vi "Common Device Queue Messenger.vi"(2 "Common Action":T1=enum."Open Front Panel", 7 "Notifier Name":string="Not a Name", 13 "Specific Action":string="No Action") -> (8 "Notifier Name":string)   [LabVIEW 2016]
uses:
  Common Device Controls/Common Device Actions.ctl
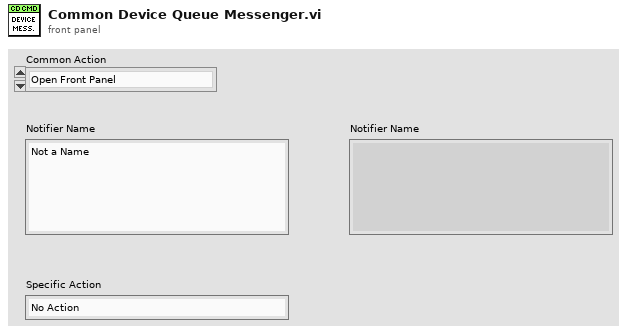
[diagram p1: front panel]
types:
  T1 = typedef "Common Device Actions.ctl" = enum16{"Specific Action", "Open Front Panel", "Close Front Panel", "Quit", "Quit All"}
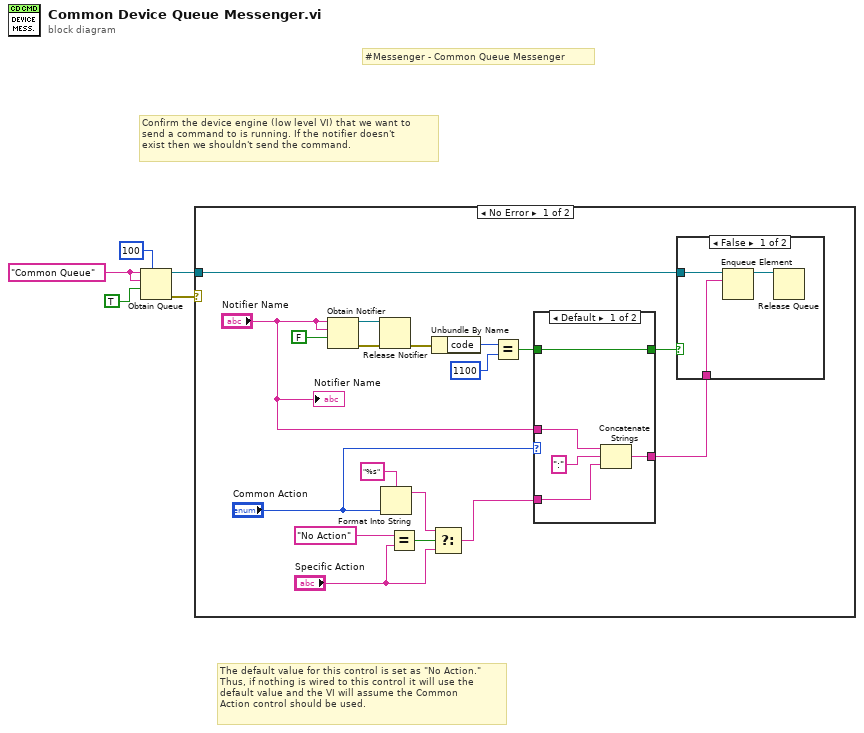
[diagram p0: block diagram]
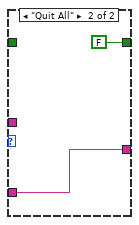
[diagram p3: hidden frame]
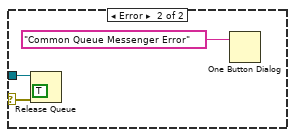
[diagram p4: hidden frame]
diagram:
  w1 = "Common Queue" ("Unique Notifier Name")
  # "Confirm the device engine (low level VI) that we want to\nsend a command to is running. If the notifier doesn't\nexist then we shouldn't send the command."
  # "The default value for this control is set as \"No Action.\"\nThus, if nothing is wired to this control it will use the\ndefault value and the VI will assume the Common\nAction control should be used."
  # "#Messenger - Common Queue Messenger"
  n1 = Obtain Queue(max queue size (-1, unlimited)=100, name (unnamed)=w1, element data type=w1, create if not found? (T)=TRUE) -> (queue out=w5:refnum<queue>, error out=w4:errorcluster)  [unwired: 1 in, 1 out]
  n2 = case shown="No Error" w4 {
    selector: w4 -> [_ w35]
    tunnel: w5 -> [w10 w37]
    frame No Error {
      n3 = Obtain Notifier(name (unnamed)="Notifier Name", notification data type="Notifier Name", create if not found? (T)=FALSE) -> (notifier out=w21:refnum<notifier>, error out=w22:errorcluster)  [unwired: 1 in, 1 out]
      n4 = Release Notifier(notifier=w21, error in (no error)=w22) -> (error out=w23:errorcluster)  [unwired: 1 in, 2 out]
      n5 = Format Into String(format string="%s", "Common Action") -> (resulting string=w16:string)  [unwired: 2 in, 1 out]
      n6 = Equal?(x="No Action" ("Unique Notifier Name"), y="Specific Action") -> (x = y?=w15:bool)
      n7 = Unbundle By Name(w23) -> ("code"=w20:i32)
      n8 = Select(t=w16, s=w15, f="Specific Action") -> (s? t:f=w12:string)
      n9 = Equal?(x=w20, y=1100) -> (x = y?=w7:bool)
      n10 = case shown="Default" "Common Action" {
        tunnel: [w31 w33] -> w9
        tunnel: w12 -> [w29 w33]
        tunnel: "Notifier Name" -> [w28 _]
        tunnel: [w27 FALSE] -> w6
        tunnel: w7 -> [w27 _]
        frame Default {
          n11 = Concatenate Strings(w28, ":" ("string"), w29) -> (w31:string)
        }
        frame "Quit All" {
        }
      }
      n12 = case shown="False" w6 {
        tunnel: w10 -> [w25 _]
        tunnel: w9 -> [w24 _]
        frame False {
          n13 = Enqueue Element(queue=w25, element=w24) -> (queue out=w26:refnum<queue>)  [unwired: 2 in, 2 out]
          n14 = Release Queue(queue=w26) -> ()  [unwired: 2 in, 3 out]
        }
        frame True {
          # "Notifier doesn't exist.\nDon't send a\ncommand"
        }
      }
      "Notifier Name" <- "Notifier Name"
    }
    frame Error {
      n15 = Release Queue(queue=w37, force destroy? (F)=TRUE, error in (no error)=w35) -> ()  [unwired: 3 out]
      n16 = One Button Dialog(message="Common Queue Messenger Error") -> ()  [unwired: 1 in, 1 out]
    }
  }
